vi "Handle Failure Action.vi"(6 "Connection Info":T1, 8 "error in (no error)":errorcluster, 9 "Created New":bool, 10 "Assert FA SEQ":refnum<queue>, 11 "Assert Message in":T3) -> (0 "error out":errorcluster, 3 "Assert Message out":T3)   [LabVIEW 2016, in "Assert API Components.lvlib" / "Log Assert Core.lvlib"]
doc: "If an assert fails then get the current information from the single element queue for the assert failure action, and then calls the appropriate class for the failure action."
uses:
  Log Assert Core.lvlib
  Message Data.ctl
  Failure Actions.ctl
  VI References.ctl
  <vilib>/NI/STM/TCP/TCP Connection Info.ctl
  <vilib>/NI/STM/SubVIs/MetaDataElement.ctl
  <vilib>/NI/STM/TCP/TCP Read Options.ctl
  Failure Actions/Abort Application/Abort Application.lvclass
  D:/Work/Projects/actor_assert_api/Core/Assert API Components/Log Assert Core Components/Failure Actions/Fail Action Base.lvclass
  Failure Actions/Log To File/Log To File.lvclass
  Failure Actions/Fail Action Base.lvclass
  Failure Actions/Pause Application/Pause Application.lvclass
  <vilib>/NI/STM/TCP/Read Message (TCP).vi
  Assert API Components.lvlib
  <vilib>/NI/STM/NI STM.lvlib
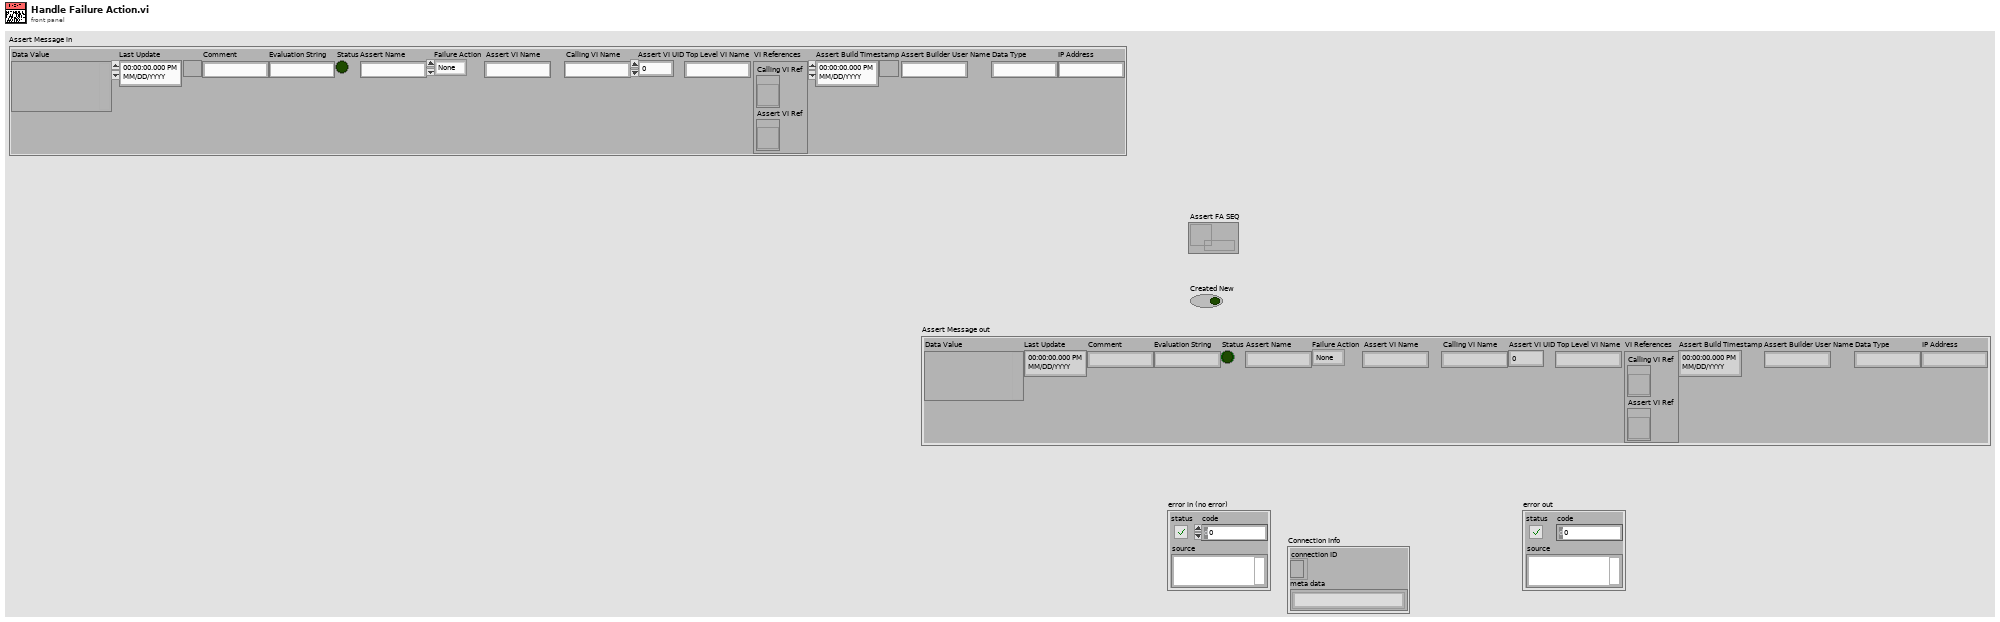
[diagram p1: front panel]
types:
  T1 = typedef "NI STM.lvlib/TCP Connection Info.ctl" = cluster{"connection ID":refnum<k5>, "meta data":T2[]}
  T2 = typedef "NI STM.lvlib/MetaDataElement.ctl" = string
  T3 = typedef "Assert API Components.lvlib/Message Data.ctl" = cluster{"Data Value":variant, "Last Update":timestamp, "Comment":string, "Evaluation String":string, "Status":bool, "Assert Name":string, "Failure Action":T4, "Assert VI Name":string, "Calling VI Name":string, "Assert VI UID":i32, "Top Level VI Name":string, "VI References":T5, "Assert Build Timestamp":timestamp, "Assert Builder User Name":string, "Data Type":string, "IP Address":string}
  T4 = typedef "Assert API Components.lvlib/Failure Actions.ctl" = enum16{"None", "Log To File", "Pause Execution", "Abort Execution"}
  T5 = typedef "Assert API Components.lvlib/VI References.ctl" = cluster{"Calling VI Ref":refnum<vi>, "Assert VI Ref":refnum<vi>}
  T6 = typedef "NI STM.lvlib/TCP Read Options.ctl" = cluster{"ignore timeout error":bool, "timeout ms (1000)":i32}
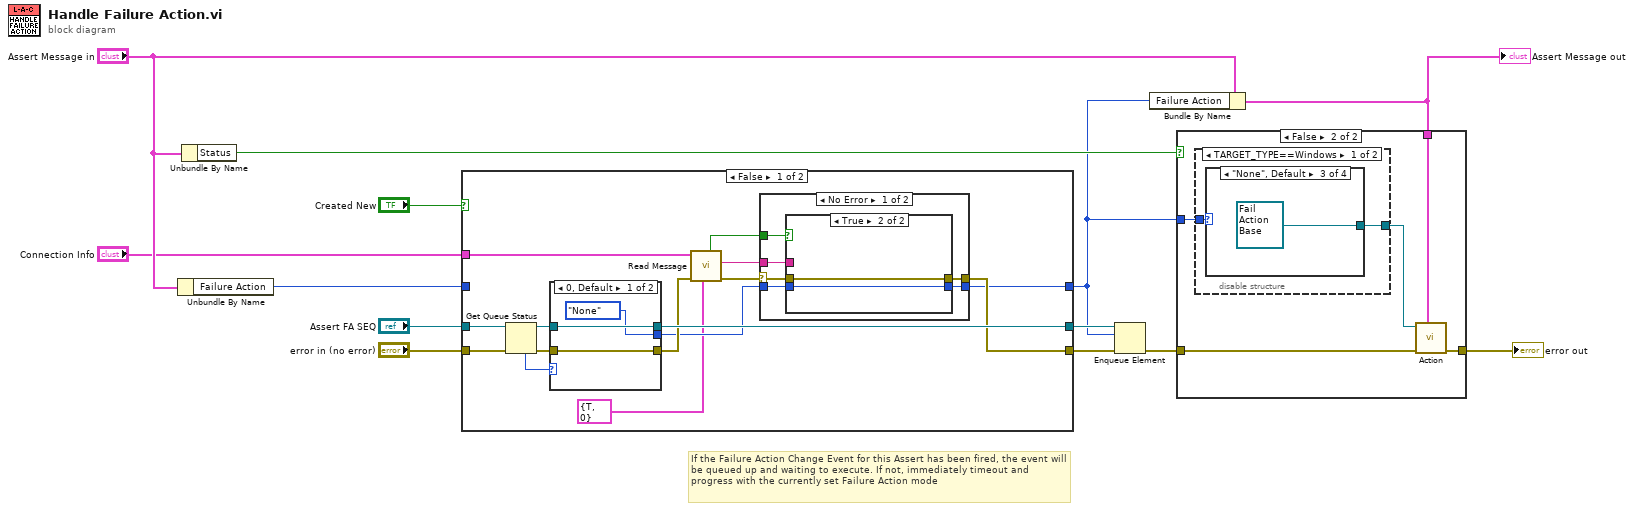
[diagram p0: block diagram]
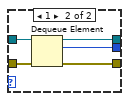
[diagram p2: hidden frame]
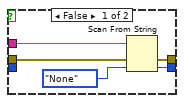
[diagram p3: hidden frame]
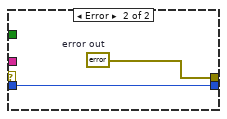
[diagram p4: hidden frame]
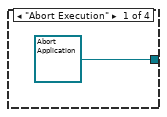
[diagram p7: hidden frame]
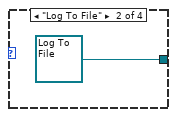
[diagram p8: hidden frame]
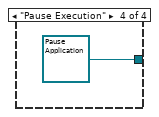
[diagram p9: hidden frame]
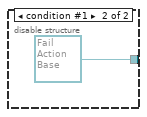
[diagram p10: hidden frame]
diagram:
  # "If the Failure Action Change Event for this Assert has been fired, the event will be queued up and waiting to execute. If not, immediately timeout and progress with the currently set Failure Action mode"
  n1 = Unbundle By Name("Assert Message in") -> ("Failure Action"=w10:T4)
  n2 = Unbundle By Name("Assert Message in") -> ("Status"=w9:bool)
  n3 = case shown="False" "Created New" {
    tunnel: [w21 w52] -> w6
    tunnel: "Connection Info" -> [w20 _]
    tunnel: "Assert FA SEQ" -> [w17 w53]
    tunnel: "error in (no error)" -> [w28 w54]
    tunnel: [w24 w54] -> w12
    tunnel: [w27 w53] -> w11
    tunnel: w10 -> [_ w52]
    frame False {
      n4 = Get Queue Status(queue=w17, error in (no error)=w28) -> (queue out=w16:refnum<queue>, error out=w18:errorcluster, # elements in queue=w15:i32)  [unwired: 1 in, 5 out]
      n5 = case shown="0, Default" w15 {
        tunnel: [w31 w36] -> w27
        tunnel: [w30 w35] -> w26
        tunnel: [Failure_Actions."None" ("Default Failure Action") w34] -> w23
        tunnel: w18 -> [w30 w33]
        tunnel: w16 -> [w31 w32]
        frame 0, Default {
        }
        frame 1 {
          n6 = Dequeue Element(queue=w32, error in (no error)=w33) -> (queue out=w36:refnum<queue>, element=w34:T4, error out=w35:errorcluster)  [unwired: 1 in, 1 out]
        }
      }
      n7 = call-poly <vilib>:"Read Message.vi"("options"=T6 {"ignore timeout error"=TRUE, "timeout ms (1000)"=0}, "error in"=w26, "connection info in"=w20) -> ("error out"=w25:errorcluster, "data string"=w22:string, "timed out?"=w14:bool)  [unwired: 3 in, 3 out]
      n8 = case shown="No Error" w25 {
        selector: w25 -> [w42 _]
        tunnel: [w39 w51] -> w21
        tunnel: [w41 w50] -> w24
        tunnel: w23 -> [w37 w51]
        tunnel: w22 -> [w40 _]
        tunnel: w14 -> [w38 _]
        frame No Error {
          n9 = case shown="True" w38 {
            tunnel: w42 -> [w47 w48]
            tunnel: [w46 w48] -> w41
            tunnel: w40 -> [w45 _]
            tunnel: [w44 w49] -> w39
            tunnel: w37 -> [_ w49]
            frame False {
              n10 = Scan From String(input string=w45, error in=w47, default 1=Failure_Actions."None" ("Default Failure Action")) -> (error out=w46:errorcluster, output 1=w44:T4)  [unwired: 2 in, 2 out]
            }
            frame True {
            }
          }
        }
        frame Error {
          w50 = errorcluster {"status"=FALSE, "code"=0, "source"=""}  # error out
        }
      }
    }
    frame True {
      # "Takes the default failure action on the first call but thereafter looks in the SEQ"
    }
  }
  n11 = Enqueue Element(queue=w11, element=w6, error in (no error)=w12) -> (error out=w5:errorcluster)  [unwired: 1 in, 2 out]
  n12 = Bundle By Name(cluster="Assert Message in", "Failure Action"=w6) -> (w4:T3)
  "Assert Message out" <- w4
  n13 = case shown="False" w9 {
    tunnel: w6 -> [_ w60]
    tunnel: w5 -> [w55 w59]
    tunnel: w4 -> [_ w57]
    tunnel: [w55 w56] -> w3
    frame True {
      # "Assert passed - no action"
    }
    frame False {
      n14 = disable-structure shown="TARGET_TYPE==Windows" {
        disable-tunnel: w60 -> [w62 _]
        disable-tunnel: [w61 refnum<class "Fail Action Base.lvclass"> refnum ("Assert API Components.lvlib:Log Assert Core.lvlib:Fail Action Base.lvclass")] -> w58
        frame condition #0 (active) {
          n15 = case shown="\"None\", Default" w62 {
            tunnel: [refnum<class "Abort Application.lvclass"> refnum ("Assert API Components.lvlib:Log Assert Core.lvlib:Abort Application.lvclass") refnum<class "Log To File.lvclass"> refnum ("Assert API Components.lvlib:Log Assert Core.lvlib:Log To File.lvclass") refnum<class "Fail Action Base.lvclass"> refnum ("Assert API Components.lvlib:Log Assert Core.lvlib:Fail Action Base.lvclass") refnum<class "Pause Application.lvclass"> refnum ("Assert API Components.lvlib:Log Assert Core.lvlib:Pause Application.lvclass")] -> w61
            frame "Abort Execution" {
            }
            frame "Log To File" {
            }
            frame "None", Default {
            }
            frame "Pause Execution" {
            }
          }
        }
        frame condition #1 {
        }
      }
      n16 = call-dynamic "Action.vi"("Assert Message"=w57, "error in (no error)"=w59, "Fail Action Base in"=w58) -> ("error out"=w56:errorcluster)  [unwired: 8 in]
    }
  }
  "error out" <- w3
